vi "Config - Update.vi"(8 "error in (no error)":errorcluster, 11 "Config Records":T1[](array[typedef])) -> (0 "error out":errorcluster, 3 "Config Records":T1[](array[typedef]))   [LabVIEW 2017]
doc: "Provide update operation for configuration database process.\n[Covers: SD5]"
uses:
  Controls/Config Record.ctl
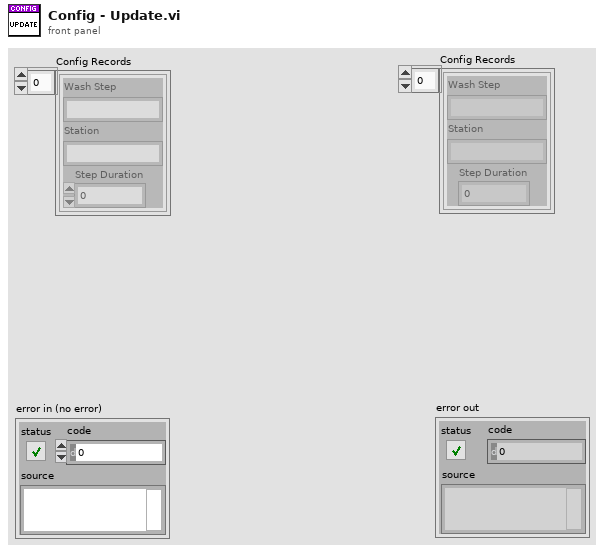
[diagram p1: front panel]
types:
  T1 = typedef "Config Record.ctl" = cluster{"Wash Step":string, "Station":string, "Step Duration":u32}
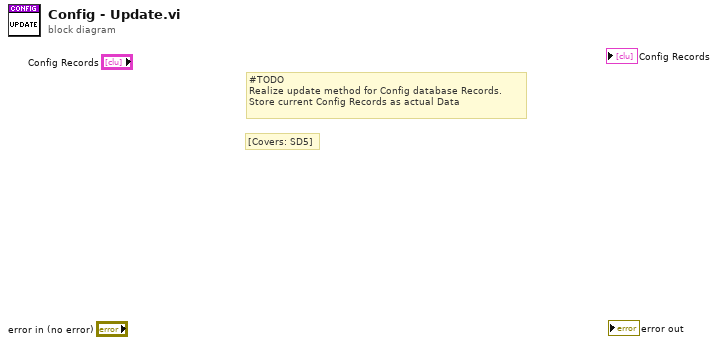
[diagram p0: block diagram]
diagram:
  # "[Covers: SD5]"
  # "#TODO\nRealize update method for Config database Records.\nStore current Config Records as actual Data"
